vi "Autonomous Independent.vi"() -> ()   [LabVIEW 2015]
doc: "This VI is called when autonomous begins, and will automatically be terminated when autonomous ends. You can carry out timed or sensor driven robot movement independently without needing to return to the caller."
uses:
  <vilib>/Rock Robotics/Network Tables/NT Read String.vi
  SubSystems/References/Refnums.vi
  Robot Global Data.vi
panel:
  out "Position":dbl
  out "Temporary Center":dbl
  # "Be sure to right-click and choose Data Operations>>Make Current Value default if you want to save the array values with the VI"
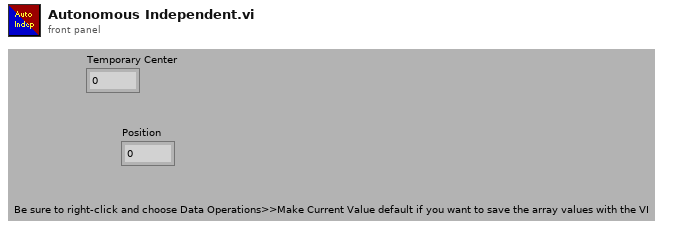
[diagram p1: front panel]
types:
  T1 = typedef "WPI_MotorControlDeviceRef.ctl" = cluster{"DeviceStatus":errorcluster, "Type":T2, "PWM":cluster{"PWM Channel":T3, "DeadBand":T4}, "CAN":cluster{"Device Number":u8, "Control Mode":T5, "Semaphore":T6, "Max Vout":dbl, "TalonSRX Control Mode":T7}, "Invert":bool}
  T2 = typedef "WPI_MotorControlType.ctl" = enum16{"PWM", "CAN", "CANTalonSRX"}
  T3 = typedef "FPGA_DIOPWMChannel.ctl" = enum8{"PWM 0", "PWM 1", "PWM 2", "PWM 3", "PWM 4", "PWM 5", "PWM 6", "PWM 7", "PWM 8", "PWM 9", "PWM MXP 0", "PWM MXP 1", "PWM MXP 2", "PWM MXP 3", "PWM MXP 4", "PWM MXP 5", "PWM MXP 6", "PWM MXP 7", "PWM MXP 8", "PWM MXP 9", "Invalid"}
  T4 = typedef "WPI_PWMDeadband.ctl" = cluster{"Name":string, "maxPositivePwm":i32, "minPositivePwm":i32, "centerPwm":i32, "maxNegativePwm":i32, "minNegativePwm":i32, "angularRange":u16}
  T5 = typedef "WPI_CANJaguar_ControlMode.ctl" = enum8{"Percent VBus", "Current", "Speed", "Position", "Voltage"}
  T6 = typedef "Semaphore RefNum" = refnum<k1>
  T7 = typedef "WPI_CANTalonSRX_APIControlMode.ctl" = enum8{"Percent VBus", "Speed", "Position", "Slave", "Unchanged / Invalid", "Voltage Compensation", "Current", "Motion Profile"}
  T8 = typedef "Relevant Data.ctl" = cluster{"Area":dbl, "CH Area":dbl, "BR Width":dbl, "BR Height":dbl, "BR Left":dbl, "BR Right":dbl}
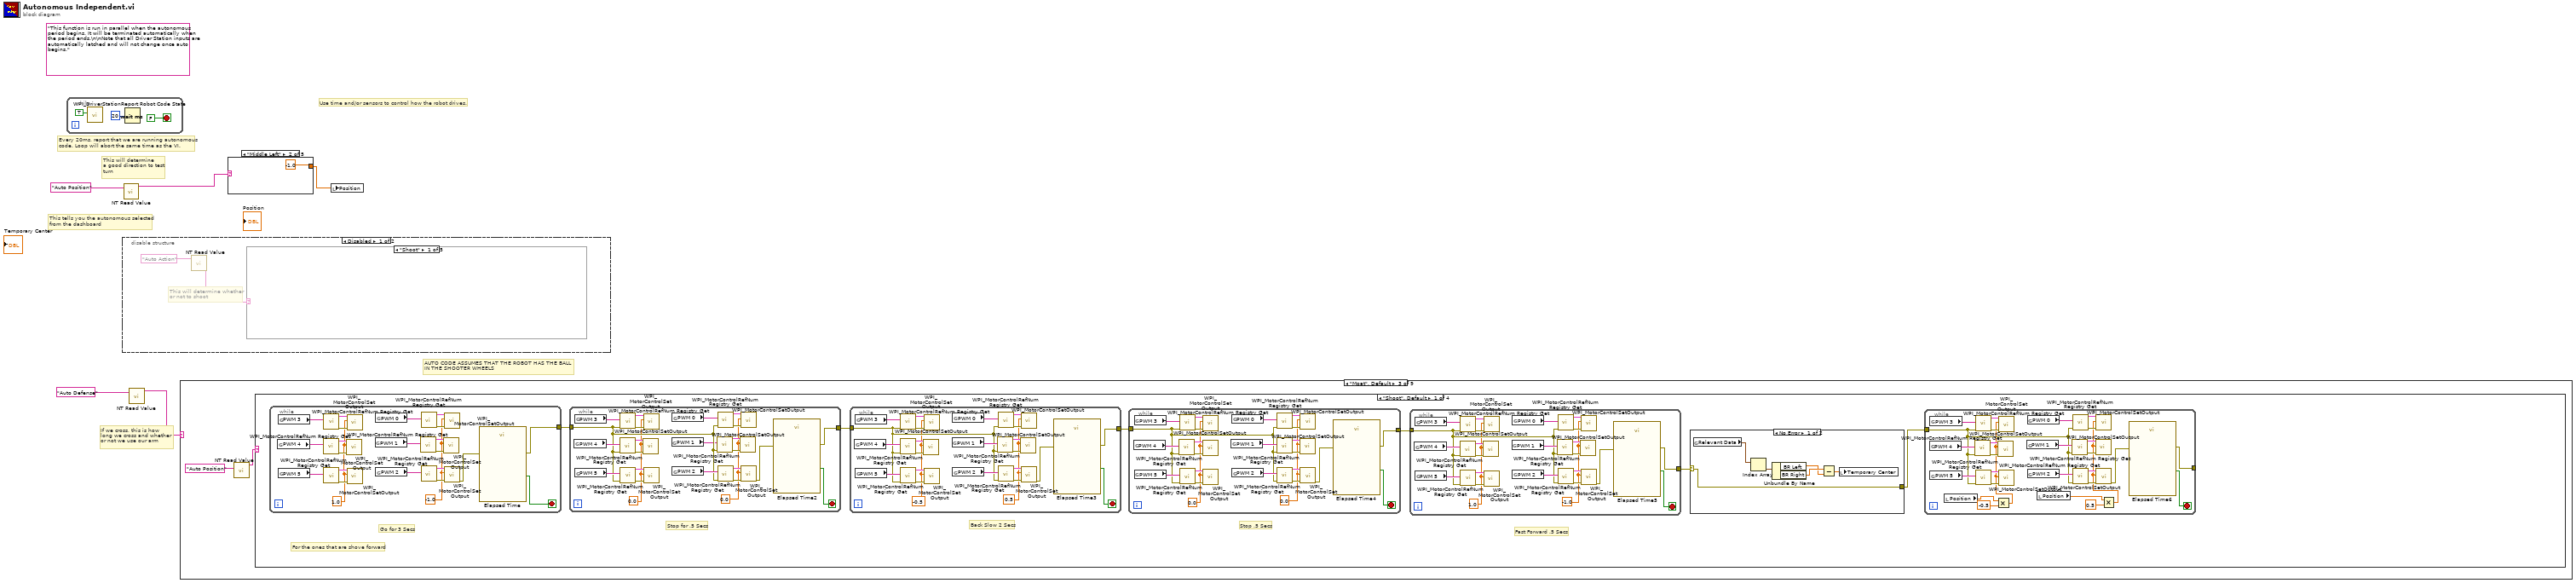
[diagram p0: block diagram]
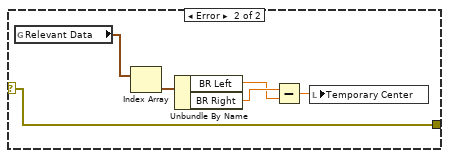
[diagram p9: hidden frame]
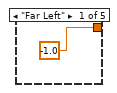
[diagram p19: hidden frame]
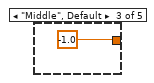
[diagram p20: hidden frame]
diagram:
  (unwired) "This function is run in parallel when the autonomous period begins. It will be terminated automatically when the period ends.\n\nNote that all Driver Station inputs are automatically latched and will not change once auto begins."
  # "AUTO CODE ASSUMES THAT THE ROBOT HAS THE BALL\nIN THE SHOOTER WHEELS"
  # "If we cross, this is how\nlong we cross and whether \nor not we use our arm"
  # "This will determine\na good direction to test\nturn"
  # "This tells you the autonomous selected\nfrom the dashboard"
  # "Every 20ms, report that we are running autonomous\ncode. Loop will abort the same time as the VI."
  # "Use time and/or sensors to control how the robot drives."
  n1 = while {
    stop <- FALSE stop-if-true
    n2 = call <vilib>:"WPI_DriverStationReport Robot Code State.vi"("Autonomous"=TRUE) -> ()  [unwired: 10 in, 1 out]
    n3 = Wait (ms)(milliseconds to wait=u32 20) -> ()  [unwired: 1 out]
  }
  n4 = disable-structure shown="Disabled" {
    frame Disabled {
      # "This will determine whether\nor not to shoot"
      n5 = call-poly <vilib>:"NT Read Value.vi"("Name"="Auto Action") -> ("String"=w9:string)  [unwired: 9 in, 1 out]
      n6 = case shown="\"Shoot\"" w9 {
        frame "Shoot" {
        }
        frame "Cross Defense" {
        }
        frame "Up to Line" {
        }
        frame "Get Ball" {
        }
        frame "Disabled" {
        }
      }
    }
    frame Enabled {
    }
  }
  n7 = call-poly <vilib>:"NT Read Value.vi"("Name"="Auto Position") -> ("String"=w4:string)  [unwired: 9 in, 1 out]
  n8 = call-poly <vilib>:"NT Read Value.vi"("Name"="Auto Defense") -> ("String"=w3:string)  [unwired: 9 in, 1 out]
  n9 = case shown="\"Moat\", Default" w3 {
    frame "Portcullis" {
    }
    frame "Cheval de Frise" {
    }
    frame "Moat", Default {
      n10 = call-poly <vilib>:"NT Read Value.vi"("Name"="Auto Position") -> ("String"=w11:string)  [unwired: 9 in, 1 out]
      n11 = case shown="\"Shoot\", Default" w11 {
        frame "Shoot", Default {
          # "Fast Forward .5 Secs"
          # "Stop .5 Secs"
          # "Back Slow 2 Secs"
          # "Stop for .5 Secs"
          # "Go for 3 Secs"
          # "For the ones that are shove forward"
          n12 = while {
            tunnel: [w155] -> w18
            stop <- w157 stop-if-true
            w158 = 1.0
            w159 = -1.0
            n13 = global read "Refnums.vi" "PWM 4"() -> (w163:string)
            n14 = global read "Refnums.vi" "PWM 3"() -> (w162:string)
            n15 = global read "Refnums.vi" "PWM 5"() -> (w168:string)
            n16 = call <vilib>:"WPI_MotorControlRefNum Registry Get.vi"("refnum name"=w163) -> ("error out"=w165:errorcluster, "MotorControlDevRef"=w164:T1)  [unwired: 9 in]
            n17 = call <vilib>:"WPI_MotorControlRefNum Registry Get.vi"("refnum name"=w162) -> ("error out"=w160:errorcluster, "MotorControlDevRef"=w161:T1)  [unwired: 9 in]
            n18 = call <vilib>:"WPI_MotorControlRefNum Registry Get.vi"("refnum name"=w168) -> ("error out"=w166:errorcluster, "MotorControlDevRef"=w167:T1)  [unwired: 9 in]
            n19 = call <vilib>:"WPI_MotorControlSetOutput.vi"("error in (no error)"=w165, "Output"=w158, "MotorControlDevRef"=w164) -> ()  [unwired: 6 in, 3 out]
            n20 = call <vilib>:"WPI_MotorControlSetOutput.vi"("error in (no error)"=w160, "Output"=w158, "MotorControlDevRef"=w161) -> ()  [unwired: 6 in, 3 out]
            n21 = call <vilib>:"WPI_MotorControlSetOutput.vi"("error in (no error)"=w166, "Output"=w158, "MotorControlDevRef"=w167) -> ()  [unwired: 6 in, 3 out]
            n22 = global read "Refnums.vi" "PWM 1"() -> (w174:string)
            n23 = global read "Refnums.vi" "PWM 0"() -> (w175:string)
            n24 = global read "Refnums.vi" "PWM 2"() -> (w169:string)
            n25 = call <vilib>:"WPI_MotorControlRefNum Registry Get.vi"("refnum name"=w174) -> ("error out"=w172:errorcluster, "MotorControlDevRef"=w173:T1)  [unwired: 9 in]
            n26 = call <vilib>:"WPI_MotorControlRefNum Registry Get.vi"("refnum name"=w175) -> ("error out"=w177:errorcluster, "MotorControlDevRef"=w176:T1)  [unwired: 9 in]
            n27 = call <vilib>:"WPI_MotorControlRefNum Registry Get.vi"("refnum name"=w169) -> ("error out"=w171:errorcluster, "MotorControlDevRef"=w170:T1)  [unwired: 9 in]
            n28 = call <vilib>:"WPI_MotorControlSetOutput.vi"("error in (no error)"=w172, "Output"=w159, "MotorControlDevRef"=w173) -> ()  [unwired: 6 in, 3 out]
            n29 = call <vilib>:"WPI_MotorControlSetOutput.vi"("error in (no error)"=w177, "Output"=w159, "MotorControlDevRef"=w176) -> ()  [unwired: 6 in, 3 out]
            n30 = call <vilib>:"WPI_MotorControlSetOutput.vi"("error in (no error)"=w171, "Output"=w159, "MotorControlDevRef"=w170) -> ("error out"=w156:errorcluster)  [unwired: 6 in, 2 out]
            n31 = call "Elapsed Time"("error in (no error)"=w156) -> ("Time has Elapsed"=w157:bool, "error out"=w155:errorcluster)  [unwired: 11 in, 6 out]
          }
          n32 = while {
            tunnel: w18 -> [w137]
            tunnel: [w132] -> w17
            stop <- w133 stop-if-true
            w136 = 0.0
            w135 = 0.0
            n33 = global read "Refnums.vi" "PWM 4"() -> (w151:string)
            n34 = global read "Refnums.vi" "PWM 3"() -> (w152:string)
            n35 = global read "Refnums.vi" "PWM 5"() -> (w146:string)
            n36 = call <vilib>:"WPI_MotorControlRefNum Registry Get.vi"("error in (no error)"=w137, "refnum name"=w151) -> ("error out"=w149:errorcluster, "MotorControlDevRef"=w150:T1)  [unwired: 8 in]
            n37 = call <vilib>:"WPI_MotorControlRefNum Registry Get.vi"("error in (no error)"=w137, "refnum name"=w152) -> ("error out"=w154:errorcluster, "MotorControlDevRef"=w153:T1)  [unwired: 8 in]
            n38 = call <vilib>:"WPI_MotorControlRefNum Registry Get.vi"("error in (no error)"=w137, "refnum name"=w146) -> ("error out"=w148:errorcluster, "MotorControlDevRef"=w147:T1)  [unwired: 8 in]
            n39 = call <vilib>:"WPI_MotorControlSetOutput.vi"("error in (no error)"=w149, "Output"=w136, "MotorControlDevRef"=w150) -> ()  [unwired: 6 in, 3 out]
            n40 = call <vilib>:"WPI_MotorControlSetOutput.vi"("error in (no error)"=w154, "Output"=w136, "MotorControlDevRef"=w153) -> ()  [unwired: 6 in, 3 out]
            n41 = call <vilib>:"WPI_MotorControlSetOutput.vi"("error in (no error)"=w148, "Output"=w136, "MotorControlDevRef"=w147) -> ()  [unwired: 6 in, 3 out]
            n42 = global read "Refnums.vi" "PWM 1"() -> (w131:string)
            n43 = global read "Refnums.vi" "PWM 0"() -> (w140:string)
            n44 = global read "Refnums.vi" "PWM 2"() -> (w145:string)
            n45 = call <vilib>:"WPI_MotorControlRefNum Registry Get.vi"("error in (no error)"=w137, "refnum name"=w131) -> ("error out"=w142:errorcluster, "MotorControlDevRef"=w141:T1)  [unwired: 8 in]
            n46 = call <vilib>:"WPI_MotorControlRefNum Registry Get.vi"("error in (no error)"=w137, "refnum name"=w140) -> ("error out"=w138:errorcluster, "MotorControlDevRef"=w139:T1)  [unwired: 8 in]
            n47 = call <vilib>:"WPI_MotorControlRefNum Registry Get.vi"("error in (no error)"=w137, "refnum name"=w145) -> ("error out"=w143:errorcluster, "MotorControlDevRef"=w144:T1)  [unwired: 8 in]
            n48 = call <vilib>:"WPI_MotorControlSetOutput.vi"("error in (no error)"=w142, "Output"=w135, "MotorControlDevRef"=w141) -> ()  [unwired: 6 in, 3 out]
            n49 = call <vilib>:"WPI_MotorControlSetOutput.vi"("error in (no error)"=w138, "Output"=w135, "MotorControlDevRef"=w139) -> ()  [unwired: 6 in, 3 out]
            n50 = call <vilib>:"WPI_MotorControlSetOutput.vi"("error in (no error)"=w143, "Output"=w135, "MotorControlDevRef"=w144) -> ("error out"=w134:errorcluster)  [unwired: 6 in, 2 out]
            n51 = call "Elapsed Time2"("error in (no error)"=w134) -> ("Time has Elapsed"=w133:bool, "error out"=w132:errorcluster)  [unwired: 11 in, 6 out]
          }
          n52 = while {
            tunnel: w17 -> [w112]
            tunnel: [w107] -> w16
            stop <- w108 stop-if-true
            w111 = -0.5
            w110 = 0.5
            n53 = global read "Refnums.vi" "PWM 4"() -> (w127:string)
            n54 = global read "Refnums.vi" "PWM 3"() -> (w128:string)
            n55 = global read "Refnums.vi" "PWM 5"() -> (w122:string)
            n56 = call <vilib>:"WPI_MotorControlRefNum Registry Get.vi"("error in (no error)"=w112, "refnum name"=w127) -> ("error out"=w125:errorcluster, "MotorControlDevRef"=w126:T1)  [unwired: 8 in]
            n57 = call <vilib>:"WPI_MotorControlRefNum Registry Get.vi"("error in (no error)"=w112, "refnum name"=w128) -> ("error out"=w130:errorcluster, "MotorControlDevRef"=w129:T1)  [unwired: 8 in]
            n58 = call <vilib>:"WPI_MotorControlRefNum Registry Get.vi"("error in (no error)"=w112, "refnum name"=w122) -> ("error out"=w124:errorcluster, "MotorControlDevRef"=w123:T1)  [unwired: 8 in]
            n59 = call <vilib>:"WPI_MotorControlSetOutput.vi"("error in (no error)"=w125, "Output"=w111, "MotorControlDevRef"=w126) -> ()  [unwired: 6 in, 3 out]
            n60 = call <vilib>:"WPI_MotorControlSetOutput.vi"("error in (no error)"=w130, "Output"=w111, "MotorControlDevRef"=w129) -> ()  [unwired: 6 in, 3 out]
            n61 = call <vilib>:"WPI_MotorControlSetOutput.vi"("error in (no error)"=w124, "Output"=w111, "MotorControlDevRef"=w123) -> ()  [unwired: 6 in, 3 out]
            n62 = global read "Refnums.vi" "PWM 1"() -> (w116:string)
            n63 = global read "Refnums.vi" "PWM 0"() -> (w115:string)
            n64 = global read "Refnums.vi" "PWM 2"() -> (w121:string)
            n65 = call <vilib>:"WPI_MotorControlRefNum Registry Get.vi"("error in (no error)"=w112, "refnum name"=w116) -> ("error out"=w118:errorcluster, "MotorControlDevRef"=w117:T1)  [unwired: 8 in]
            n66 = call <vilib>:"WPI_MotorControlRefNum Registry Get.vi"("error in (no error)"=w112, "refnum name"=w115) -> ("error out"=w113:errorcluster, "MotorControlDevRef"=w114:T1)  [unwired: 8 in]
            n67 = call <vilib>:"WPI_MotorControlRefNum Registry Get.vi"("error in (no error)"=w112, "refnum name"=w121) -> ("error out"=w119:errorcluster, "MotorControlDevRef"=w120:T1)  [unwired: 8 in]
            n68 = call <vilib>:"WPI_MotorControlSetOutput.vi"("error in (no error)"=w118, "Output"=w110, "MotorControlDevRef"=w117) -> ()  [unwired: 6 in, 3 out]
            n69 = call <vilib>:"WPI_MotorControlSetOutput.vi"("error in (no error)"=w113, "Output"=w110, "MotorControlDevRef"=w114) -> ()  [unwired: 6 in, 3 out]
            n70 = call <vilib>:"WPI_MotorControlSetOutput.vi"("error in (no error)"=w119, "Output"=w110, "MotorControlDevRef"=w120) -> ("error out"=w109:errorcluster)  [unwired: 6 in, 2 out]
            n71 = call "Elapsed Time3"("error in (no error)"=w109) -> ("Time has Elapsed"=w108:bool, "error out"=w107:errorcluster)  [unwired: 11 in, 6 out]
          }
          n72 = while {
            tunnel: w16 -> [w88]
            tunnel: [w83] -> w15
            stop <- w84 stop-if-true
            w87 = 0.0
            w86 = 0.0
            n73 = global read "Refnums.vi" "PWM 4"() -> (w103:string)
            n74 = global read "Refnums.vi" "PWM 3"() -> (w104:string)
            n75 = global read "Refnums.vi" "PWM 5"() -> (w98:string)
            n76 = call <vilib>:"WPI_MotorControlRefNum Registry Get.vi"("error in (no error)"=w88, "refnum name"=w103) -> ("error out"=w101:errorcluster, "MotorControlDevRef"=w102:T1)  [unwired: 8 in]
            n77 = call <vilib>:"WPI_MotorControlRefNum Registry Get.vi"("error in (no error)"=w88, "refnum name"=w104) -> ("error out"=w106:errorcluster, "MotorControlDevRef"=w105:T1)  [unwired: 8 in]
            n78 = call <vilib>:"WPI_MotorControlRefNum Registry Get.vi"("error in (no error)"=w88, "refnum name"=w98) -> ("error out"=w100:errorcluster, "MotorControlDevRef"=w99:T1)  [unwired: 8 in]
            n79 = call <vilib>:"WPI_MotorControlSetOutput.vi"("error in (no error)"=w101, "Output"=w87, "MotorControlDevRef"=w102) -> ()  [unwired: 6 in, 3 out]
            n80 = call <vilib>:"WPI_MotorControlSetOutput.vi"("error in (no error)"=w106, "Output"=w87, "MotorControlDevRef"=w105) -> ()  [unwired: 6 in, 3 out]
            n81 = call <vilib>:"WPI_MotorControlSetOutput.vi"("error in (no error)"=w100, "Output"=w87, "MotorControlDevRef"=w99) -> ()  [unwired: 6 in, 3 out]
            n82 = global read "Refnums.vi" "PWM 1"() -> (w92:string)
            n83 = global read "Refnums.vi" "PWM 0"() -> (w91:string)
            n84 = global read "Refnums.vi" "PWM 2"() -> (w97:string)
            n85 = call <vilib>:"WPI_MotorControlRefNum Registry Get.vi"("error in (no error)"=w88, "refnum name"=w92) -> ("error out"=w94:errorcluster, "MotorControlDevRef"=w93:T1)  [unwired: 8 in]
            n86 = call <vilib>:"WPI_MotorControlRefNum Registry Get.vi"("error in (no error)"=w88, "refnum name"=w91) -> ("error out"=w89:errorcluster, "MotorControlDevRef"=w90:T1)  [unwired: 8 in]
            n87 = call <vilib>:"WPI_MotorControlRefNum Registry Get.vi"("error in (no error)"=w88, "refnum name"=w97) -> ("error out"=w95:errorcluster, "MotorControlDevRef"=w96:T1)  [unwired: 8 in]
            n88 = call <vilib>:"WPI_MotorControlSetOutput.vi"("error in (no error)"=w94, "Output"=w86, "MotorControlDevRef"=w93) -> ()  [unwired: 6 in, 3 out]
            n89 = call <vilib>:"WPI_MotorControlSetOutput.vi"("error in (no error)"=w89, "Output"=w86, "MotorControlDevRef"=w90) -> ()  [unwired: 6 in, 3 out]
            n90 = call <vilib>:"WPI_MotorControlSetOutput.vi"("error in (no error)"=w95, "Output"=w86, "MotorControlDevRef"=w96) -> ("error out"=w85:errorcluster)  [unwired: 6 in, 2 out]
            n91 = call "Elapsed Time4"("error in (no error)"=w85) -> ("Time has Elapsed"=w84:bool, "error out"=w83:errorcluster)  [unwired: 11 in, 6 out]
          }
          n92 = while {
            tunnel: w15 -> [w64]
            tunnel: [w59] -> w14
            stop <- w60 stop-if-true
            w63 = 1.0
            w62 = -1.0
            n93 = global read "Refnums.vi" "PWM 4"() -> (w79:string)
            n94 = global read "Refnums.vi" "PWM 3"() -> (w80:string)
            n95 = global read "Refnums.vi" "PWM 5"() -> (w74:string)
            n96 = call <vilib>:"WPI_MotorControlRefNum Registry Get.vi"("error in (no error)"=w64, "refnum name"=w79) -> ("error out"=w77:errorcluster, "MotorControlDevRef"=w78:T1)  [unwired: 8 in]
            n97 = call <vilib>:"WPI_MotorControlRefNum Registry Get.vi"("error in (no error)"=w64, "refnum name"=w80) -> ("error out"=w82:errorcluster, "MotorControlDevRef"=w81:T1)  [unwired: 8 in]
            n98 = call <vilib>:"WPI_MotorControlRefNum Registry Get.vi"("error in (no error)"=w64, "refnum name"=w74) -> ("error out"=w76:errorcluster, "MotorControlDevRef"=w75:T1)  [unwired: 8 in]
            n99 = call <vilib>:"WPI_MotorControlSetOutput.vi"("error in (no error)"=w77, "Output"=w63, "MotorControlDevRef"=w78) -> ()  [unwired: 6 in, 3 out]
            n100 = call <vilib>:"WPI_MotorControlSetOutput.vi"("error in (no error)"=w82, "Output"=w63, "MotorControlDevRef"=w81) -> ()  [unwired: 6 in, 3 out]
            n101 = call <vilib>:"WPI_MotorControlSetOutput.vi"("error in (no error)"=w76, "Output"=w63, "MotorControlDevRef"=w75) -> ()  [unwired: 6 in, 3 out]
            n102 = global read "Refnums.vi" "PWM 1"() -> (w68:string)
            n103 = global read "Refnums.vi" "PWM 0"() -> (w67:string)
            n104 = global read "Refnums.vi" "PWM 2"() -> (w73:string)
            n105 = call <vilib>:"WPI_MotorControlRefNum Registry Get.vi"("error in (no error)"=w64, "refnum name"=w68) -> ("error out"=w70:errorcluster, "MotorControlDevRef"=w69:T1)  [unwired: 8 in]
            n106 = call <vilib>:"WPI_MotorControlRefNum Registry Get.vi"("error in (no error)"=w64, "refnum name"=w67) -> ("error out"=w65:errorcluster, "MotorControlDevRef"=w66:T1)  [unwired: 8 in]
            n107 = call <vilib>:"WPI_MotorControlRefNum Registry Get.vi"("error in (no error)"=w64, "refnum name"=w73) -> ("error out"=w71:errorcluster, "MotorControlDevRef"=w72:T1)  [unwired: 8 in]
            n108 = call <vilib>:"WPI_MotorControlSetOutput.vi"("error in (no error)"=w70, "Output"=w62, "MotorControlDevRef"=w69) -> ()  [unwired: 6 in, 3 out]
            n109 = call <vilib>:"WPI_MotorControlSetOutput.vi"("error in (no error)"=w65, "Output"=w62, "MotorControlDevRef"=w66) -> ()  [unwired: 6 in, 3 out]
            n110 = call <vilib>:"WPI_MotorControlSetOutput.vi"("error in (no error)"=w71, "Output"=w62, "MotorControlDevRef"=w72) -> ("error out"=w61:errorcluster)  [unwired: 6 in, 2 out]
            n111 = call "Elapsed Time5"("error in (no error)"=w61) -> ("Time has Elapsed"=w60:bool, "error out"=w59:errorcluster)  [unwired: 11 in, 6 out]
          }
          n112 = case shown="No Error" w14 {
            selector: w14 -> [w47 w53]
            tunnel: [w47 w53] -> w13
            frame No Error {
              n113 = global read "Robot Global Data.vi" "Relevant Data"() -> (w52:T8[])
              n114 = Index Array(array=w52) -> (element=w51:T8)  [unwired: 1 in]
              n115 = Unbundle By Name(w51) -> ("BR Left"=w49:dbl, "BR Right"=w50:dbl)
              n116 = Subtract(x=w50, y=w49) -> (x-y=w48:dbl)
              n117 = local write "Temporary Center"(w48) -> ()
            }
            frame Error {
              n118 = global read "Robot Global Data.vi" "Relevant Data"() -> (w58:T8[])
              n119 = Index Array(array=w58) -> (element=w57:T8)  [unwired: 1 in]
              n120 = Unbundle By Name(w57) -> ("BR Left"=w55:dbl, "BR Right"=w56:dbl)
              n121 = Subtract(x=w56, y=w55) -> (x-y=w54:dbl)
              n122 = local write "Temporary Center"(w54) -> ()
            }
          }
          n123 = while {
            tunnel: w13 -> [w28]
            tunnel: [w25] -> _
            stop <- w26 stop-if-true
            n124 = global read "Refnums.vi" "PWM 4"() -> (w43:string)
            n125 = global read "Refnums.vi" "PWM 3"() -> (w44:string)
            n126 = global read "Refnums.vi" "PWM 5"() -> (w38:string)
            n127 = local read "Position"() -> (w23:dbl)
            n128 = call <vilib>:"WPI_MotorControlRefNum Registry Get.vi"("error in (no error)"=w28, "refnum name"=w43) -> ("error out"=w41:errorcluster, "MotorControlDevRef"=w42:T1)  [unwired: 8 in]
            n129 = call <vilib>:"WPI_MotorControlRefNum Registry Get.vi"("error in (no error)"=w28, "refnum name"=w44) -> ("error out"=w46:errorcluster, "MotorControlDevRef"=w45:T1)  [unwired: 8 in]
            n130 = call <vilib>:"WPI_MotorControlRefNum Registry Get.vi"("error in (no error)"=w28, "refnum name"=w38) -> ("error out"=w40:errorcluster, "MotorControlDevRef"=w39:T1)  [unwired: 8 in]
            n131 = Multiply(x=w23, y=-0.5) -> (x*y=w21:dbl)
            n132 = call <vilib>:"WPI_MotorControlSetOutput.vi"("error in (no error)"=w41, "Output"=w21, "MotorControlDevRef"=w42) -> ()  [unwired: 6 in, 3 out]
            n133 = call <vilib>:"WPI_MotorControlSetOutput.vi"("error in (no error)"=w46, "Output"=w21, "MotorControlDevRef"=w45) -> ()  [unwired: 6 in, 3 out]
            n134 = call <vilib>:"WPI_MotorControlSetOutput.vi"("error in (no error)"=w40, "Output"=w21, "MotorControlDevRef"=w39) -> ()  [unwired: 6 in, 3 out]
            n135 = global read "Refnums.vi" "PWM 1"() -> (w32:string)
            n136 = global read "Refnums.vi" "PWM 0"() -> (w31:string)
            n137 = global read "Refnums.vi" "PWM 2"() -> (w37:string)
            n138 = local read "Position"() -> (w20:dbl)
            n139 = call <vilib>:"WPI_MotorControlRefNum Registry Get.vi"("error in (no error)"=w28, "refnum name"=w32) -> ("error out"=w34:errorcluster, "MotorControlDevRef"=w33:T1)  [unwired: 8 in]
            n140 = call <vilib>:"WPI_MotorControlRefNum Registry Get.vi"("error in (no error)"=w28, "refnum name"=w31) -> ("error out"=w29:errorcluster, "MotorControlDevRef"=w30:T1)  [unwired: 8 in]
            n141 = call <vilib>:"WPI_MotorControlRefNum Registry Get.vi"("error in (no error)"=w28, "refnum name"=w37) -> ("error out"=w35:errorcluster, "MotorControlDevRef"=w36:T1)  [unwired: 8 in]
            n142 = Multiply(x=w20, y=0.5) -> (x*y=w19:dbl)
            n143 = call <vilib>:"WPI_MotorControlSetOutput.vi"("error in (no error)"=w34, "Output"=w19, "MotorControlDevRef"=w33) -> ()  [unwired: 6 in, 3 out]
            n144 = call <vilib>:"WPI_MotorControlSetOutput.vi"("error in (no error)"=w29, "Output"=w19, "MotorControlDevRef"=w30) -> ()  [unwired: 6 in, 3 out]
            n145 = call <vilib>:"WPI_MotorControlSetOutput.vi"("error in (no error)"=w35, "Output"=w19, "MotorControlDevRef"=w36) -> ("error out"=w27:errorcluster)  [unwired: 6 in, 2 out]
            n146 = call "Elapsed Time6"("error in (no error)"=w27) -> ("Time has Elapsed"=w26:bool, "error out"=w25:errorcluster)  [unwired: 11 in, 6 out]
          }
        }
        frame "Cross Defense" {
        }
        frame "Up to Line" {
        }
        frame "Disabled" {
        }
      }
    }
    frame "Ramparts" {
    }
    frame "Drawbridge" {
    }
    frame "Sally Port" {
    }
    frame "Rock Wall" {
    }
    frame "Rough Terrain" {
    }
    frame "Low Bar" {
    }
  }
  n147 = case shown="\"Middle Left\"" w4 {
    tunnel: [-1.0 -1.0 -1.0 1.0 1.0] -> w1
    frame "Far Left" {
    }
    frame "Middle Left" {
    }
    frame "Middle", Default {
    }
    frame "Middle Right" {
    }
    frame "Far Right" {
    }
  }
  n148 = local write "Position"(w1) -> ()
